vi "init.vi"(8 "error in":errorcluster, 10 "TBM module configuration in":refnum<class "TBM module configuration.lvclass">, 11 "Sequencer Module runtime in":refnum<class "Sequencer Module runtime.lvclass">) -> (0 "error out":errorcluster, 1 "data allocations":T1, 2 "execution settings":T4, 3 "Sequencer Module runtime out":refnum<class "Sequencer Module runtime.lvclass">)   [LabVIEW 2015, in "Sequencer Module runtime.lvclass"]
doc: "Provides an interface for initializing a module at runtime. While this interface performs no operations, a child should provide an override which may open any necessary references or sessions, allocate necessary memory, and perform any final configuration validataion before providing the full configuration <b>execution data</b> to the calling process."
uses:
  Sequencer Module runtime.lvclass
  <vilib>/NI/Tag Bus Module Framework/module configuration/TBM module configuration.lvclass
  <vilib>/NI/Tag Bus Module Framework/runtime/execution settings.ctl
  <vilib>/NI/Tag Bus Module Framework/channel/data tables.ctl
  <vilib>/NI/Tag Bus/dictionary/data dictionary.lvclass
  <vilib>/NI/Tag Bus/dictionary table pair.ctl
  <vilib>/NI/Tag Bus/table/data table.ctl
  configuration/Sequencer Module configuration.lvclass
  Sequencer State Enum.ctl
  classes/Result Processor/Execution/ResultProcessor.lvclass
  configuration/Sequencer Module configuration.lvclass/Sequencer Module configuration.ctl
  Sequencer Module runtime.lvclass/Sequencer Module runtime.ctl
  configuration/Read Lines.vi
  classes/Result Processor/Config/ResultProcessor Config.lvclass
  classes/Sequence/Config/Sequence Config.lvclass
  <vilib>/NI/Tag Bus Module Framework/channel/TBM channel.lvclass
  <vilib>/NI/Tag Bus Module Framework/runtime/TBM module execution interface.lvclass
  <vilib>/NI/Tag Bus/tag bus.lvlib
  <vilib>/NI/Tag Bus/table/data table.lvlib
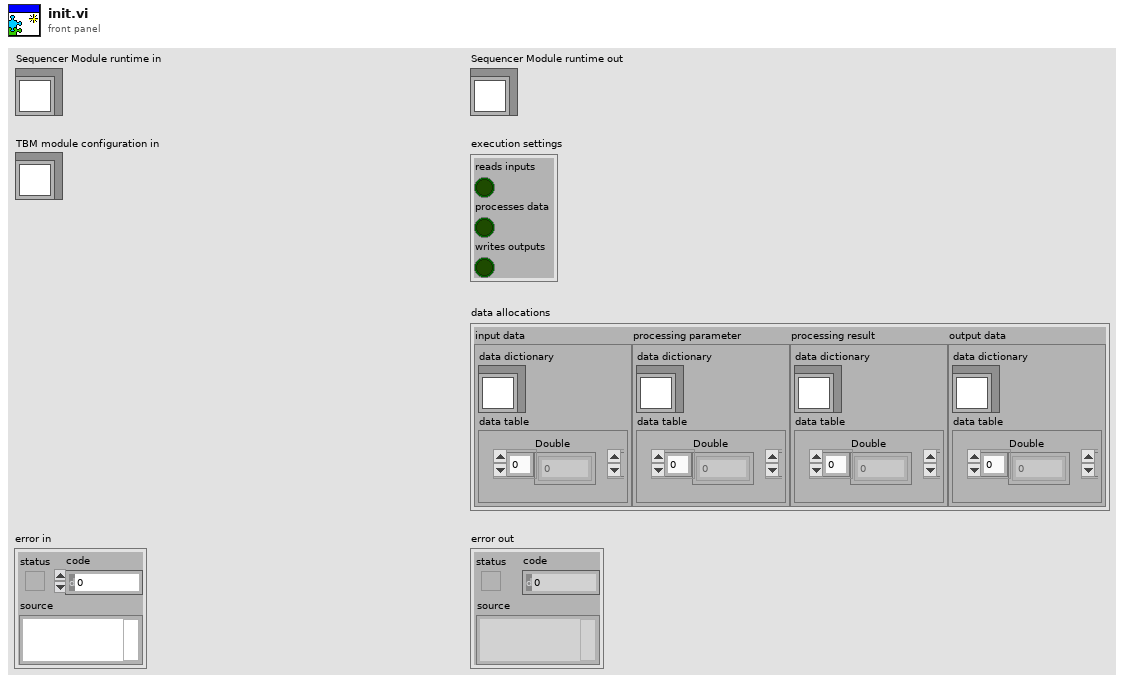
[diagram p1: front panel]
types:
  T1 = typedef "TBM channel.lvclass/data tables.ctl" = cluster{"input data":T2, "processing parameter":T2, "processing result":T2, "output data":T2}
  T2 = typedef "tag bus.lvlib/dictionary table pair.ctl" = cluster{"data dictionary":refnum<class "data dictionary.lvclass">, "data table":T3}
  T3 = typedef "tag bus.lvlib/data table.lvlib/data table.ctl" = cluster{"Double":dbl[], "Single":sgl[], "I64":i64[], "I32":i32[], "I16":i16[], "I8":i8[], "U64":u64[], "U32":u32[], "U16":u16[], "U8":u8[], "Boolean":bool[], "String":string[], "Array of Double":cluster{"DBL Array":dbl[]}[], "Array of Single":cluster{"SGL Array":sgl[]}[], "Array of I64":cluster{"I64 Array":i64[]}[], "Array of I32":cluster{"I32 Array":i32[]}[], "Array of I16":cluster{"I16 Array":i16[]}[], "Array of I8":cluster{"I8 Array":i8[]}[], "Array of U64":cluster{"U64 Array":u64[]}[], "Array of U32":cluster{"U32 Array":u32[]}[], "Array of U16":cluster{"U16 Array":u16[]}[], "Array of U8":cluster{"U8 Array":u8[]}[], "Array of Boolean":cluster{"Boolean Array":bool[]}[], "Array of String":cluster{"String Array":string[]}[]}
  T4 = typedef "TBM module execution interface.lvclass/execution settings.ctl" = cluster{"reads inputs":bool, "processes data":bool, "writes outputs":bool}
  T5 = typedef "Sequencer Module runtime.lvclass/Sequencer State Enum.ctl" = enum16{"Idle", "Paused", "Start Sequence", "Run Sequence", "CleanUp Sequence", "Generate Report"}
  T6 = typedef "Sequencer Module configuration.lvclass/Line.ctl" = cluster{"Sequence":refnum<class "Sequence Config.lvclass">}
  T7 = cluster{"Station ID":i32, "Station SN":i32, "DUT SN":i32, "DUT Info":i32}
  T8 = typedef "Sequencer Module runtime.lvclass/Sequencer State Index.ctl" = cluster{"Sequencer State":i32, "Active Sequence Name":i32, "Active Sequence Index":i32, "Active Step":i32, "Active Step State":i32, "Active Step UI Alias":i32}
  T9 = typedef "Sequencer Module runtime.lvclass/Sequencer Control Index.ctl" = cluster{"Start":i32, "Change Sequence":i32, "New Sequence":i32, "Pause":i32}
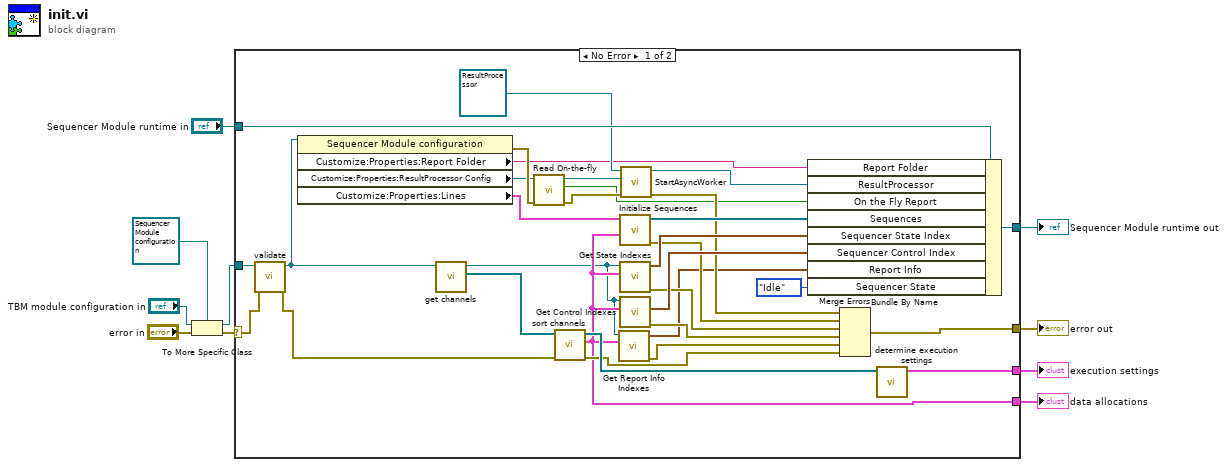
[diagram p0: block diagram]
diagram:
  n1 = To More Specific Class(target class=refnum<class "Sequencer Module configuration.lvclass"> refnum ("Synchronous module configuration"), reference="TBM module configuration in", error in="error in") -> (specific class reference=w9:refnum<class "Sequencer Module configuration.lvclass">, error out=w10:errorcluster)
  n2 = case shown="No Error" w10 {
    selector: w10 -> [w39 w43]
    tunnel: w9 -> [w38 _]
    tunnel: "Sequencer Module runtime in" -> [w37 w44]
    tunnel: [w36 w44] -> w4
    tunnel: [w27 w43] -> w3
    tunnel: [w14 _] -> w1
    tunnel: [w42 _] -> w2
    frame No Error {
      n3 = call-dynamic "validate.vi"("error in"=w39, "Sequencer Module configuration in"=w38) -> ("error out"=w40:errorcluster, "Sequencer Module configuration out"=w35:refnum<class "Sequencer Module configuration.lvclass">)  [unwired: 8 in]
      n4 = property class="Sequencer Module configuration"(reference=w35) -> (error out=w19:errorcluster, "Customize:Properties:Report Folder"=w15:string, "Customize:Properties:ResultProcessor Config"=w16:refnum<class "ResultProcessor Config.lvclass">, "Customize:Properties:Lines"=w34:T6[])  [unwired: 1 in, 1 out]
      n5 = call-dynamic "get channels.vi"("Sequencer Module configuration in"=w35) -> ("channels"=w32:refnum<class "TBM channel.lvclass">[], "Sequencer Module configuration out"=w13:refnum<class "Sequencer Module configuration.lvclass">)  [unwired: 9 in]
      n6 = call-dynamic "Read On-the-fly.vi"("error in (no error)"=w19, "ResultProcessor Config in"=w16) -> ("error out"=w18:errorcluster, "On-the-fly?"=w17:bool, "ResultProcessor Config out"=w20:refnum<class "ResultProcessor Config.lvclass">)  [unwired: 7 in]
      n7 = call <vilib>:"sort channels.vi"("error in"=w40, "channels in"=w32) -> ("error out"=w28:errorcluster, "data allocations"=w14:T1, "channels out"=w41:refnum<class "TBM channel.lvclass">[])  [unwired: 7 in]
      n8 = call "Get Report Info Indexes.vi"("data allocations"=w14, "Sequencer Module configuration in"=w13) -> ("error out"=w12:errorcluster, "Cluster"=w11:T7)  [unwired: 8 in]
      n9 = call "Initialize Sequences.vi"("data allocations"=w14, "Customize:Properties:Lines"=w34) -> ("error out"=w26:errorcluster, "Array"=w33:refnum<class "Sequence.lvclass">[])  [unwired: 8 in]
      n10 = call "Get State Indexes.vi"("data allocations"=w14, "Sequencer Module configuration in"=w13) -> ("error out"=w25:errorcluster, "Sequencer State Index"=w31:T8)  [unwired: 8 in]
      n11 = call "Get Control Indexes.vi"("data allocations"=w14, "Sequencer Module configuration in"=w13) -> ("error out"=w24:errorcluster, "Sequencer Control Index"=w29:T9)  [unwired: 8 in]
      n12 = call "StartAsyncWorker.vi"("error in (no error)"=w18, "ResultProcessor Config.lvclass"=w20, "ResultProcessor in"=refnum<class "ResultProcessor.lvclass"> refnum ("ResultProcessor.lvclass")) -> ("error out"=w21:errorcluster, "ResultProcessor out"=w22:refnum<class "ResultProcessor.lvclass">)  [unwired: 7 in]
      n13 = Bundle By Name(cluster=w37, "Report Folder"=w15, "ResultProcessor"=w22, "On the Fly Report"=w17, "Sequences"=w33, "Sequencer State Index"=w31, "Sequencer Control Index"=w29, "Report Info"=w11, "Sequencer State"=Sequencer_State_Enum."Idle" ("Sequencer State.Sequencer State")) -> (w36:refnum<class "Sequencer Module runtime.lvclass">)
      n14 = Merge Errors(w21, w26, w25, w24, w12, w28) -> (w27:errorcluster)
      n15 = call <vilib>:"determine execution settings.vi"("channels"=w41) -> ("execution settings"=w42:T4)  [unwired: 10 in]
    }
    frame Error {
    }
  }
  "error out" <- w3
  "Sequencer Module runtime out" <- w4
  "execution settings" <- w2
  "data allocations" <- w1
